vi "calc wait time sub.vi"(1 "mm to go":dbl, 2 "set speed (steps/s)":dbl) -> (0 "wait time":dbl)   [LabVIEW 2018]
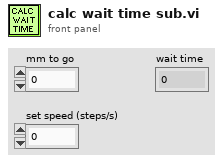
[diagram p1: front panel]
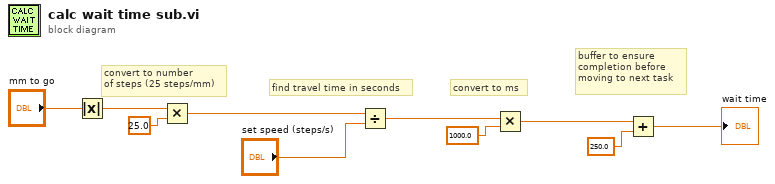
[diagram p0: block diagram]
diagram:
  # "buffer to ensure\ncompletion before\nmoving to next task"
  # "find travel time in seconds"
  # "convert to number\nof steps (25 steps/mm)"
  # "convert to ms"
  n1 = Absolute Value(x="mm to go") -> (abs(x)=w2:dbl)
  n2 = Multiply(x=w2, y=25.0) -> (x*y=w7:dbl)
  n3 = Divide(x=w7, y="set speed (steps/s)") -> (x/y=w6:dbl)
  n4 = Multiply(x=w6, y=1000.0) -> (x*y=w10:dbl)
  n5 = Add(x=w10, y=250.0) -> (x+y=→"wait time":dbl)
